vi "create_data_folders.vi"(9 "Date array":string[](array[string]), 10 "Experiment Indicator":string, 11 "username":string) -> (3 "Data Output Folder":path)   [LabVIEW 2016]
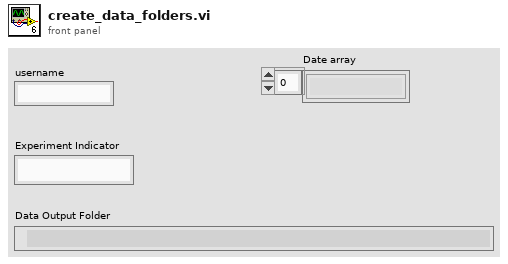
[diagram p1: front panel]
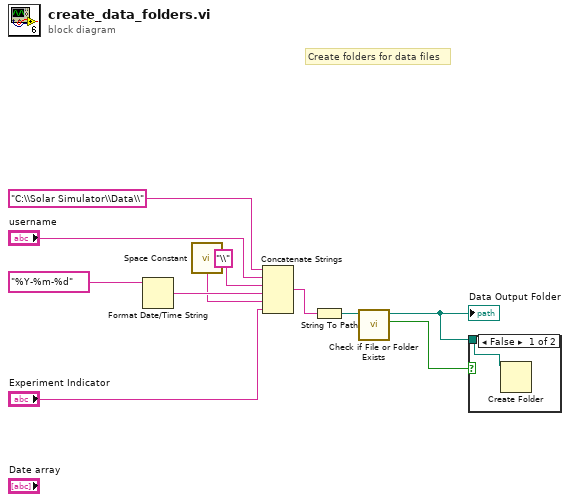
[diagram p0: block diagram]
diagram:
  # "Create folders for data files"
  n1 = Format Date/Time String(time format string (%c)="%Y-%m-%d") -> (date/time string=w4:string)  [unwired: 2 in]
  n2 = call <vilib>:"Space Constant.vi"() -> ("String"=w1:string)
  n3 = Concatenate Strings("C:\\Solar Simulator\\Data\\", "username", "\\", w4, w1, "Experiment Indicator") -> (w7:string)
  n4 = String To Path(string=w7) -> (path=w10:path)
  n5 = call <vilib>:"Check if File or Folder Exists.vi"("path"=w10) -> ("file or folder exists?"=w11:bool, "dup path"=w6:path)  [unwired: 8 in, 1 out]
  "Data Output Folder" <- w6
  n6 = case shown="False" w11 {
    tunnel: w6 -> [w12 _]
    frame False {
      n7 = Create Folder(path (use dialog)=w12) -> ()  [unwired: 2 in, 3 out]
    }
    frame True {
    }
  }
